vi "Low-Level ReadConfig.vi"(8 "error in (no error)":errorcluster, 9 "Timeout":i32=200, 10 "Command":string, 11 "Agilent DSO-X 3032A in":refnum<class "Agilent DSO-X 3032A.lvclass">) -> (0 "error out":errorcluster, 1 "Data as DBL":dbl, 2 "Data":string, 3 "Agilent DSO-X 3032A out":refnum<class "Agilent DSO-X 3032A.lvclass">)   [LabVIEW 2014, in "Agilent DSO-X 3032A.lvclass"]
uses:
  Agilent DSO-X 3032A/Agilent DSO-X 3032A.lvclass
  Agilent DSO-X 3032A/Agilent DSO-X 3032A.lvclass/Agilent DSO-X 3032A.ctl
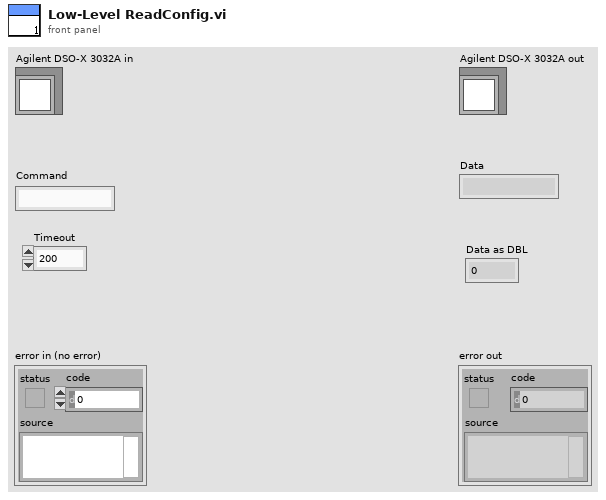
[diagram p1: front panel]
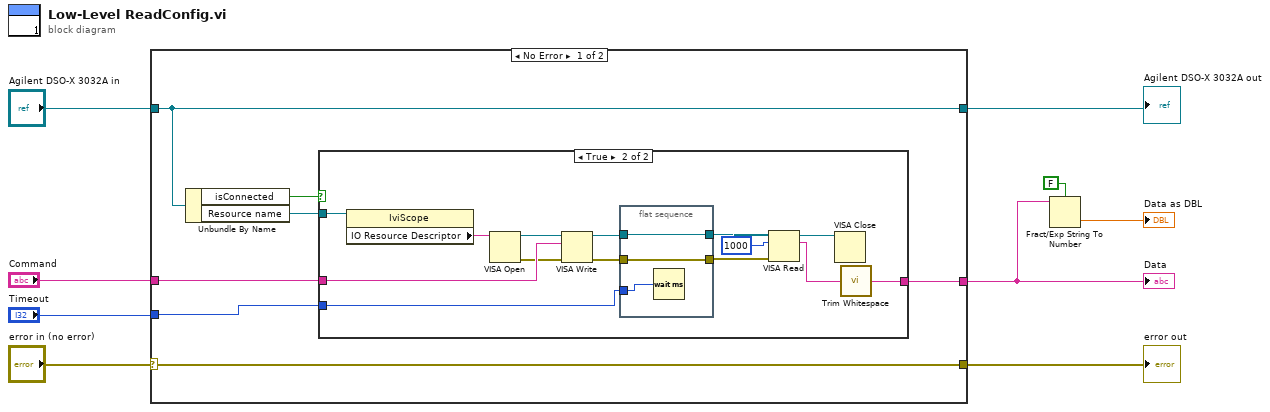
[diagram p0: block diagram]
diagram:
  n1 = case shown="No Error" "error in (no error)" {
    selector: "error in (no error)" -> [w16 w35]
    tunnel: [w16 w35] -> w8
    tunnel: [w15 w34] -> w6
    tunnel: "Agilent DSO-X 3032A in" -> [w15 w34]
    tunnel: "Command" -> [w12 _]
    tunnel: [w11 _] -> w4
    tunnel: "Timeout" -> [w10 _]
    frame No Error {
      n2 = Unbundle By Name(w15) -> ("isConnected"=w14:bool, "Resource name"=w13:refnum<k15>)
      n3 = case shown="True" w14 {
        tunnel: w13 -> [_ w25]
        tunnel: w12 -> [_ w24]
        tunnel: [_ w18] -> w11
        tunnel: w10 -> [_ w17]
        frame False {
        }
        frame True {
          n4 = property class="IviScope"(reference=w25) -> ("IO Resource Descriptor"=w26:string)  [unwired: 1 in, 2 out]
          n5 = VISA Open(VISA resource name=w26) -> (VISA resource name=w29:refnum<visa-resource-name>, error out=w22:errorcluster)  [unwired: 4 in]
          n6 = VISA Write(VISA resource name=w29, write buffer=w24, error in (no error)=w22) -> (VISA resource name out=w28:refnum<visa-resource-name>, error out=w21:errorcluster)  [unwired: 1 out]
          n7 = flat-sequence {
            tunnel: w28 -> [w33]
            tunnel: [w33] -> w27
            tunnel: w21 -> [w32]
            tunnel: [w32] -> w20
            tunnel: w17 -> [w31]
            frame #0 {
              n8 = Wait (ms)(milliseconds to wait=w31) -> ()  [unwired: 1 out]
            }
          }
          n9 = VISA Read(VISA resource name=w27, byte count=u32 1000, error in (no error)=w20) -> (VISA resource name out=w30:refnum<visa-resource-name>, read buffer=w19:string)  [unwired: 2 out]
          n10 = VISA Close(VISA resource name=w30) -> ()  [unwired: 1 in, 1 out]
          n11 = call <vilib>:"Trim Whitespace.vi"("string"=w19) -> ("trimmed string"=w18:string)  [unwired: 1 in]
        }
      }
    }
    frame Error {
    }
  }
  "error out" <- w8
  "Data" <- w4
  "Agilent DSO-X 3032A out" <- w6
  n12 = Fract/Exp String To Number(use system decimal point (T)=FALSE, string=w4) -> (number=→"Data as DBL":dbl)  [unwired: 2 in, 1 out]
